vi "DAQ_CounterTrigger_DO_AO.vi"(8 "error in (no error)":errorcluster) -> (0 "error out":errorcluster)   [LabVIEW 2025]
uses:
  SubVIs/State_Machine_Ctrl.ctl
  <vilib>/DAQmx/write.llb/DAQmx Write (Digital 1D Wfm NChan NSamp).vi
  <vilib>/DAQmx/write.llb/DAQmx Write (Analog 1D Wfm NChan NSamp).vi
  <vilib>/Waveform/DWDTOps.llb/DWDT Uncompress Digital.vi
  <vilib>/DAQmx/miscellaneous.llb/DAQmx Fill In Error Info.vi
  <vilib>/Waveform/WDTOps.llb/WDT Waveform Duration DBL.vi
  <resource>/objmgr/daqmx.rc
panel:
  out "duration":dbl
  out "AO WF":waveform(dbl)[](graph)=[{"t0"=timestamp(0 s since 1904-01-01), "dt"=0.0001, "Y"=array[18000 elements]}, {"t0"=timestamp(0 s since 1904-01-01), "dt"=0.0001, "Y"=array[18000 elements]}, {"t0"=timestamp(0 s since 1904-01-01), "dt"=0.0001, "Y"=array[18000 elements]}, {"t0"=timestamp(0 s since 1904-01-01), "dt"=0.0001, "Y"=array[18000 elements]}]
  out "DO WF":digitalwaveform[](graph)=[{"t0"=timestamp(0 s since 1904-01-01), "dt"=0.0001, "Y"={"transitions"=[], "data"=array18000x1[18000 elements]}}, {"t0"=timestamp(0 s since 1904-01-01), "dt"=0.0001, "Y"={"transitions"=[], "data"=array18000x1[18000 elements]}}, {"t0"=timestamp(0 s since 1904-01-01), "dt"=0.0001, "Y"={"transitions"=[], "data"=array18000x1[18000 elements]}}, {"t0"=timestamp(0 s since 1904-01-01), "dt"=0.0001, "Y"={"transitions"=[], "data"=array18000x1[18000 elements]}}]
  in  "AO | %":dbl[](array[slide])=[47.78761061946903, 65.48672566371681] min=0.0 max=100.0 step=1.0 scale=0.0..100.0
  in  "AO | ON/OFF":bool[](array[boolean])=[TRUE, TRUE, TRUE, TRUE]
  out "AO | Peripherals":string[](array[string])=["Laser 1", "Laser 2", "Pockels", "Z stage"]
  out "DO | Peripherals":string[](array[string])=["Laser 1", "Laser 2", "Blanking", "Camera"]
  in  "DO | ON/OFF":bool[](array[boolean])=[TRUE, TRUE, TRUE, TRUE]
  in  "Pre-activation time (s)":dbl=0.03
  in  "Start":bool
  in  "Readout time (s)":dbl=0.02
  in  "Exposure time (s)":dbl=0.05
  in  "Stop":bool
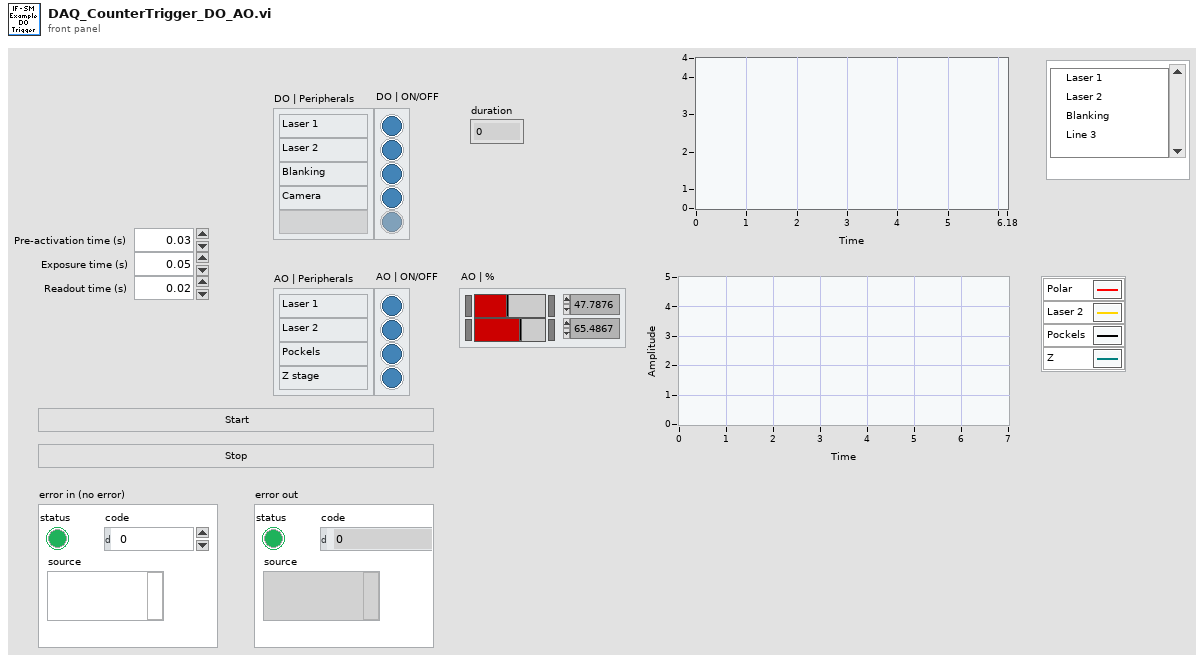
[diagram p1: front panel]
types:
  T1 = typedef "State_Machine_Ctrl.ctl" = enum16{"Initialize", "Wait for Event", "Setup_DAQ", "Create WF", "Generate WF", "Stop"}
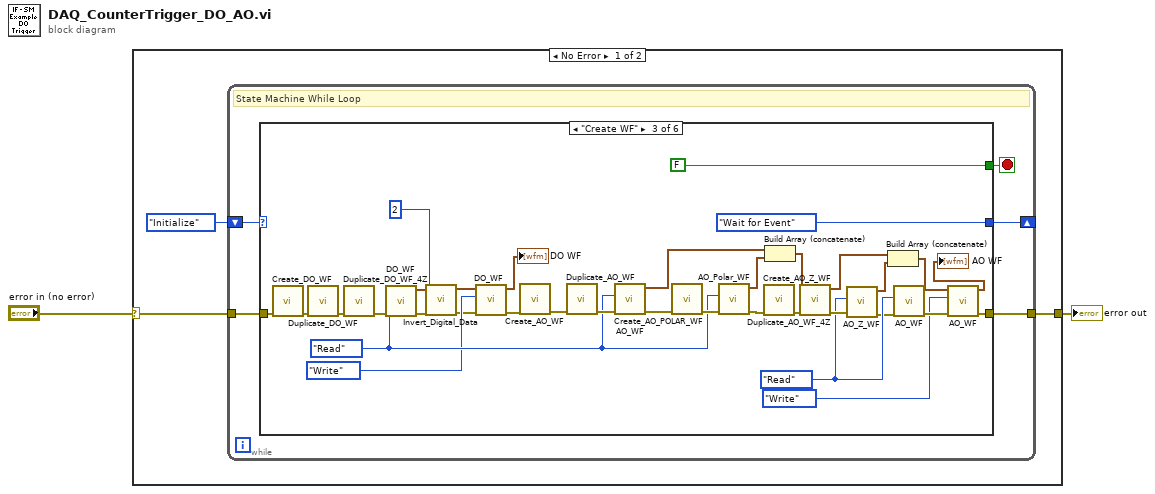
[diagram p0: block diagram]
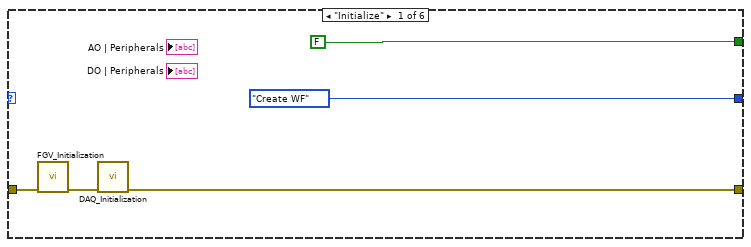
[diagram p2: hidden frame]
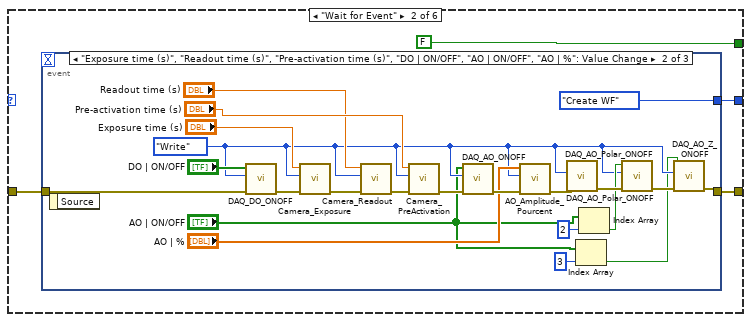
[diagram p3: hidden frame]
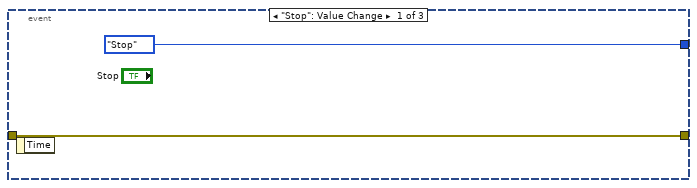
[diagram p4: hidden frame]
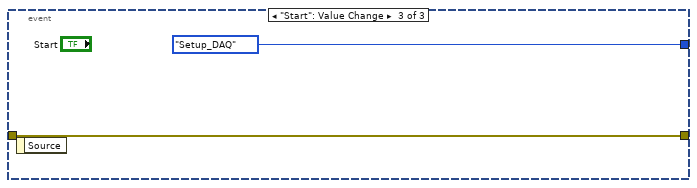
[diagram p5: hidden frame]
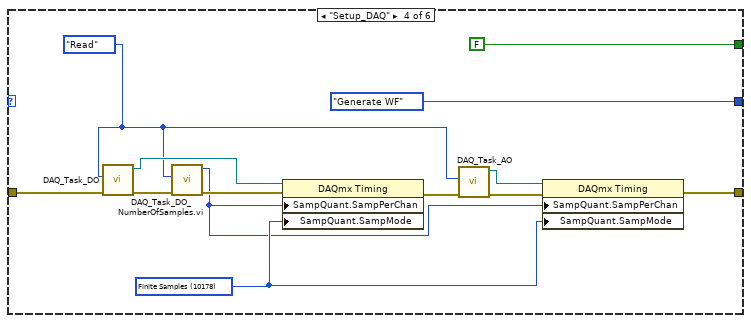
[diagram p6: hidden frame]
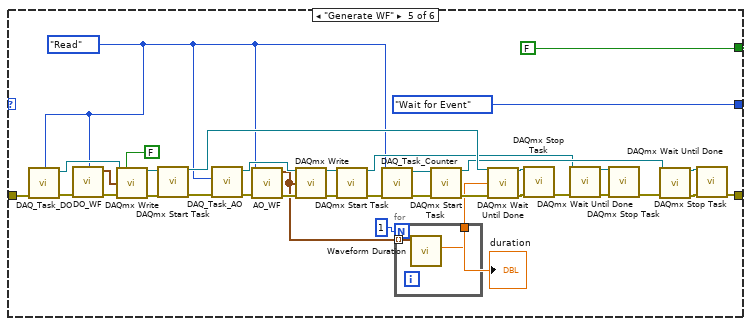
[diagram p7: hidden frame]
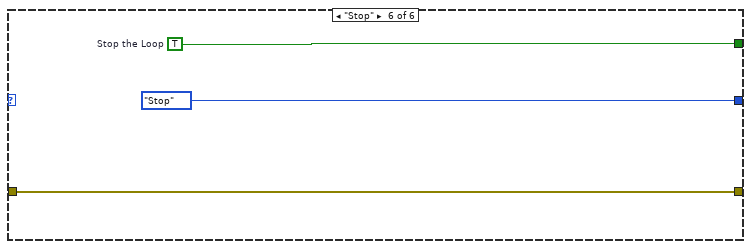
[diagram p8: hidden frame]
diagram:
  n1 = case shown="No Error" "error in (no error)" {
    selector: "error in (no error)" -> [w4 w134]
    tunnel: [w3 w134] -> w2
    frame No Error {
      n2 = while {
        shift-right: [w9] -> _
        shift-left: State_Machine_Ctrl."Initialize" ("Initial State") -> [w10]
        tunnel: w4 -> [w7]
        tunnel: [w6] -> w3
        stop <- w8 stop-if-true
        # "State Machine While Loop"
        n3 = case "State Machine Case Structure" shown="\"Create WF\"" w10 {
          tunnel: [State_Machine_Ctrl."Create WF" ("Initial State") w19 State_Machine_Ctrl."Wait for Event" ("Initial State") State_Machine_Ctrl."Generate WF" ("Initial State") State_Machine_Ctrl."Wait for Event" ("Initial State") State_Machine_Ctrl."Stop" ("Initial State")] -> w9
          tunnel: [FALSE ("Stop the Loop") FALSE ("Stop the Loop") FALSE ("Stop the Loop") FALSE ("Stop the Loop") FALSE ("Stop the Loop") w133] -> w8
          tunnel: w7 -> [w13 w17 w77 w90 w125 w131]
          tunnel: [w14 w16 w73 w87 w112 w131] -> w6
          frame "Initialize" {
            # "Initialize - In this example, the only initialization required is to specify that the next state for the state machine is \"Wait for Event\"."
            n4 = call "FGV_Initialization.vi"("error in (no error)"=w13) -> ("error out"=w12:errorcluster)  [unwired: 10 in]
            n5 = call "DAQ_Initialization.vi"("error in (no error)"=w12) -> ("error out"=w14:errorcluster)  [unwired: 10 in]
          }
          frame "Wait for Event" {
            # "Wait for Event - An Event Structure is used to monitor the user interface for events. In each frame of the Event Structure, the next state of the state machine is specified based on which button was pressed."
            n6 = event shown="[1] \"Exposure time (s)\", \"Readout time (s)\", \"Pre-activation time (s)\", \"DO | ON/OFF\", \"AO | ON/OFF\", \"AO | %\": Value Change" {
              selector: _ -> [_ _ _]
              dyn-events: _ -> [_ _ _]
              timeout: _ -> [_ _ _]
              tunnel: [State_Machine_Ctrl."Stop" ("Initial State") State_Machine_Ctrl."Create WF" ("Initial State") State_Machine_Ctrl."Setup_DAQ" ("Initial State")] -> w19
              tunnel: w17 -> [w20 w39 w44]
              tunnel: [w20 w26 w44] -> w16
              event "Stop": Value Change {
                n7 = event-data() -> ()  [unwired: 1 in, 1 out]
              }
              event "Exposure time (s)", "Readout time (s)", "Pre-activation time (s)", "DO | ON/OFF", "AO | ON/OFF", "AO | %": Value Change {
                w25 = enum16{"Init", "Write", "Read"}."Write" ("Action")
                n8 = event-data() -> ()  [unwired: 1 in, 1 out]
                n9 = call "DAQ_DO_ONOFF.vi"("error in"=w39, "Action"=w25, "DO | ON/OFF"="DO | ON/OFF") -> ("error out"=w42:errorcluster)  [unwired: 7 in, 1 out]
                n10 = call "Camera_Exposure.vi"("error in"=w42, "Action"=w25, "Exposure (s)"="Exposure time (s)") -> ("error out"=w41:errorcluster)  [unwired: 7 in, 1 out]
                n11 = call "Camera_Readout.vi"("error in"=w41, "Action"=w25, "Camera_Readout"="Readout time (s)") -> ("error out"=w40:errorcluster)  [unwired: 7 in, 1 out]
                n12 = call "Camera_PreActivation.vi"("error in"=w40, "Action"=w25, "Camera_PreActivation"="Pre-activation time (s)") -> ("error out"=w34:errorcluster)  [unwired: 7 in, 1 out]
                n13 = call "DAQ_AO_ONOFF.vi"("error in"=w34, "Action"=w25, "AO | ON/OFF"="AO | ON/OFF") -> ("error out"=w33:errorcluster)  [unwired: 7 in, 1 out]
                n14 = call "AO_Amplitude_Pourcent.vi"("error in"=w33, "Action"=w25, "AO | %"="AO | %") -> ("error out"=w31:errorcluster)  [unwired: 7 in, 1 out]
                n15 = call "DAQ_AO_Polar_ONOFF.vi"("error in"=w31, "Action"=w25) -> ("error out"=w30:errorcluster)  [unwired: 8 in, 1 out]
                n16 = Index Array(array="AO | ON/OFF", index=3) -> (element=w23:bool)
                n17 = Index Array(array="AO | ON/OFF", index=2) -> (element=w28:bool)
                n18 = call "DAQ_AO_Polar_ONOFF.vi"("error in"=w30, "Action"=w25, "ON / OFF"=w28) -> ("error out"=w27:errorcluster)  [unwired: 7 in, 1 out]
                n19 = call "DAQ_AO_Z_ONOFF.vi"("error in"=w27, "Action"=w25, "ON / OFF"=w23) -> ("error out"=w26:errorcluster)  [unwired: 7 in, 1 out]
              }
              event "Start": Value Change {
                n20 = event-data() -> ()  [unwired: 1 in, 1 out]
              }
            }
          }
          frame "Create WF" {
            w60 = enum16{"Init", "Write", "Read"}."Read" ("Action")
            w65 = enum16{"Init", "Write", "Read"}."Read" ("Action")
            n21 = call "Create_DO_WF.vi"("error in"=w77) -> ("error out"=w76:errorcluster)  [unwired: 10 in]
            n22 = call "Duplicate_DO_WF.vi"("error in"=w76) -> ("error out"=w71:errorcluster)  [unwired: 9 in, 1 out]
            n23 = call "Duplicate_DO_WF_4Z.vi"("error in"=w71) -> ("error out"=w70:errorcluster)  [unwired: 10 in]
            n24 = call "DO_WF.vi"("error in"=w70, "Action"=w65) -> ("error out"=w50:errorcluster, "Digital WF"=w48:digitalwaveform[])  [unwired: 8 in]
            n25 = call "Invert_Digital_Data.vi"("error in (no error)"=w50, "Index to invert"=2, "DO WF"=w48) -> ("error out"=w49:errorcluster, "DO WF 2"=w47:digitalwaveform[])  [unwired: 7 in]
            n26 = call "DO_WF.vi"("error in"=w49, "Action"=enum16{"Init", "Write", "Read"}."Write", "Digital WF"=w47) -> ("error out"=w53:errorcluster, "Digital WF"=→"DO WF":digitalwaveform[])  [unwired: 7 in]
            n27 = call "Create_AO_WF.vi"("error in"=w53) -> ("error out"=w67:errorcluster)  [unwired: 10 in]
            n28 = call "Duplicate_AO_WF.vi"("error in (no error)"=w67) -> ("error out"=w66:errorcluster)  [unwired: 10 in]
            n29 = call "AO_WF.vi"("error in"=w66, "Action"=w65) -> ("error out"=w64:errorcluster, "AO WF"=w69:waveform(dbl)[])  [unwired: 8 in]
            n30 = call "Create_AO_POLAR_WF.vi"("error in"=w64) -> ("error out"=w68:errorcluster)  [unwired: 10 in]
            n31 = call "AO_Polar_WF.vi"("error in"=w68, "Action"=w65) -> ("error out"=w63:errorcluster, "AO Poalr WF"=w75:waveform(dbl))  [unwired: 8 in]
            n32 = call "Create_AO_Z_WF.vi"("error in"=w63) -> ("error out"=w62:errorcluster)  [unwired: 10 in]
            n33 = Build Array (concatenate)(w69, w75) -> (w59:waveform(dbl)[])
            n34 = call "Duplicate_AO_WF_4Z.vi"("error in (no error)"=w62, "AO WF"=w59) -> ("error out"=w61:errorcluster, "AO WF 2"=w56:waveform(dbl)[])  [unwired: 8 in]
            n35 = call "AO_Z_WF.vi"("error in"=w61, "Action"=w60) -> ("error out"=w58:errorcluster, "AO Z WF"=w55:waveform(dbl))  [unwired: 8 in]
            n36 = Build Array (concatenate)(w56, w55) -> (w57:waveform(dbl)[])
            n37 = call "AO_WF.vi"("error in"=w58, "Action"=w60) -> ("error out"=w74:errorcluster)  [unwired: 8 in, 1 out]
            n38 = call "AO_WF.vi"("error in"=w74, "Action"=enum16{"Init", "Write", "Read"}."Write", "AO WF"=w57) -> ("error out"=w73:errorcluster, "AO WF"=→"AO WF":waveform(dbl)[])  [unwired: 7 in]
          }
          frame "Setup_DAQ" {
            w80 = enum16{"Init", "Write", "Read"}."Read" ("Action")
            w84 = 10178 items=["Finite Samples"=10178, "Continuous Samples"=10123, "Hardware Timed Single Point"=12522] ("SampQuant.SampMode")
            n39 = call "DAQ_Task_DO.vi"("error in"=w90, "Action"=w80) -> ("error out"=w83:errorcluster, "DAQ_Task_DO"=w89:refnum<k21>)  [unwired: 8 in]
            n40 = call "DAQ_Task_DO_NumberOfSamples.vi.vi"("error in"=w83, "Action"=w80) -> ("error out"=w82:errorcluster, "Samples"=w81:u32)  [unwired: 8 in]
            n41 = property class="DAQmx Timing"(reference=w89, error in=w82, "SampQuant.SampPerChan"=w81, "SampQuant.SampMode"=w84) -> (error out=w85:errorcluster)  [unwired: 1 out]
            n42 = call "DAQ_Task_AO.vi"("error in"=w85, "Action"=w80) -> ("error out"=w88:errorcluster, "DAQ_Task_DO"=w86:refnum<k21>)  [unwired: 8 in]
            n43 = property class="DAQmx Timing"(reference=w86, error in=w88, "SampQuant.SampPerChan"=w81, "SampQuant.SampMode"=w84) -> (error out=w87:errorcluster)  [unwired: 1 out]
          }
          frame "Generate WF" {
            w96 = enum16{"Init", "Write", "Read"}."Read" ("Action")
            n44 = call "DAQ_Task_DO.vi"("error in"=w125, "Action"=w96) -> ("error out"=w109:errorcluster, "DAQ_Task_DO"=w124:refnum<k21>)  [unwired: 8 in]
            n45 = call "DO_WF.vi"("error in"=w109, "Action"=w96) -> ("error out"=w108:errorcluster, "Digital WF"=w110:digitalwaveform[])  [unwired: 8 in]
            n46 = call-poly <vilib>:"DAQmx Write.vi"("task/channels in"=w124, "auto start"=FALSE, "data"=w110, "error in"=w108) -> ("task out"=w123:refnum<k21>, "error out"=w126:errorcluster)  [unwired: 9 in, 1 out]
            n47 = call <vilib>:"DAQmx Start Task.vi"("task/channels in"=w123, "error in"=w126) -> ("task out"=w116:refnum<k21>, "error out"=w111:errorcluster)  [unwired: 12 in]
            n48 = call "DAQ_Task_AO.vi"("error in"=w111, "Action"=w96) -> ("error out"=w103:errorcluster, "DAQ_Task_DO"=w102:refnum<k21>)  [unwired: 8 in]
            n49 = call "AO_WF.vi"("error in"=w103, "Action"=w96) -> ("error out"=w101:errorcluster, "AO WF"=w95:waveform(dbl)[])  [unwired: 8 in]
            n50 = call-poly <vilib>:"DAQmx Write.vi"("task/channels in"=w102, "data"=w95, "error in"=w101) -> ("task out"=w100:refnum<k21>, "error out"=w99:errorcluster)  [unwired: 10 in, 1 out]
            n51 = call <vilib>:"DAQmx Start Task.vi"("task/channels in"=w100, "error in"=w99) -> ("task out"=w97:refnum<k21>, "error out"=w98:errorcluster)  [unwired: 12 in]
            n52 = call "DAQ_Task_Counter.vi"("error in"=w98, "Action"=w96) -> ("error out"=w121:errorcluster, "DAQ_Task_Counter"=w122:refnum<k21>)  [unwired: 8 in]
            n53 = for {
              N: 1 -> [_]
              tunnel: w95 -> [w130] mode=indexing
              tunnel: [w129] -> w93
              n54 = call-poly <vilib>:"Waveform Duration.vi"("waveform in"=w130) -> ("duration"=w129:dbl)  [unwired: 8 in, 2 out]
            }
            "duration" <- w93
            n55 = call <vilib>:"DAQmx Start Task.vi"("task/channels in"=w122, "error in"=w121) -> ("task out"=w114:refnum<k21>, "error out"=w113:errorcluster)  [unwired: 12 in]
            n56 = call <vilib>:"DAQmx Wait Until Done.vi"("task/channels in"=w116, "timeout (sec)"=w93, "error in"=w113) -> ("task out"=w115:refnum<k21>, "error out"=w117:errorcluster)  [unwired: 11 in]
            n57 = call <vilib>:"DAQmx Stop Task.vi"("task/channels in"=w115, "error in"=w117) -> ("error out"=w106:errorcluster)  [unwired: 12 in, 1 out]
            n58 = call <vilib>:"DAQmx Wait Until Done.vi"("task/channels in"=w97, "error in"=w106) -> ("task out"=w104:refnum<k21>, "error out"=w107:errorcluster)  [unwired: 12 in]
            n59 = call <vilib>:"DAQmx Stop Task.vi"("task/channels in"=w104, "error in"=w107) -> ("error out"=w105:errorcluster)  [unwired: 12 in, 1 out]
            n60 = call <vilib>:"DAQmx Wait Until Done.vi"("task/channels in"=w114, "error in"=w105) -> ("task out"=w119:refnum<k21>, "error out"=w118:errorcluster)  [unwired: 12 in]
            n61 = call <vilib>:"DAQmx Stop Task.vi"("task/channels in"=w119, "error in"=w118) -> ("error out"=w112:errorcluster)  [unwired: 12 in, 1 out]
          }
          frame "Stop" {
            w133 = TRUE  # Stop the Loop
            # "Stop - Stop the VI. This is the only state that specifies a TRUE value for the loop conditional terminal."
          }
        }
      }
    }
    frame Error {
    }
  }
  "error out" <- w2
